vi "Big_LED_control.vi"() -> ()   [LabVIEW 2018]
uses:
  <instrlib>/niDMM/nidmm.llb/niDMM Function.ctl
  <instrlib>/niDMM/nidmm.llb/niDMM Resolution in Digits.ctl
  <instrlib>/niDCPower/nidcpower.llb/niDCPower Measurement Type.ctl
  <instrlib>/niDMM/nidmm.llb/niDMM Configure Measurement Digits.vi
  <vilib>/Instr/_visa.llb/VISA Configure Serial Port (Instr).vi
panel:
  in  "Записать":bool
  in  "Command":string="led_on"
  in  "Tab Control":enum32{"Рабочая область", "Служебная область"}(tab)
  in  "POWER":bool
  in  "Стоп":bool
  in  "Resource Name":refnum<k15>="PXI1Slot2" caption="Источник питания"
  in  "Амперметр":refnum<k15>="PXI1Slot5" caption="NI DMM 1"
  in  "V_MB, V":dbl=5.0 caption="voltage level" format="%_6p"
  in  "curlim_V_MB, A":dbl=0.3 caption="current limit" format="%_6p"
  in  "curlim_V_RESERVE, A":dbl=0.1 caption="current limit" min=0.01 format="%_6p"
  out "currentmes_V_MB, A":dbl caption="measurement" format="%_6g"
  out "currentmes_V_RESERVE, A":dbl caption="measurement" format="%_6g"
  in  "V_RESERVE, V":dbl caption="voltage level" format="%_6p"
  out "chart_2":dbl(graph)=8.556104343922883e-07
  out "chart_0":dbl(graph)=5.42616690347781e-05 caption="Waveform Chart 5"
  in  "curlim_V_LED, A":dbl=0.01 caption="current limit" min=0.01 format="%_6p"
  in  "V_LED, V":dbl=2.000000000000001 caption="voltage level" format="%_6p"
  out "chart_1":dbl(graph)=2.456762028615791e-06 caption="Waveform Chart 5"
  out "currentmes_V_LED, A":dbl caption="measurement" format="%_6g"
  in  "NI DMM 1 Current Range 3":string(combo)="1" caption="Range"
  in  "NI DMM 1 units 3":string(combo)="1000" caption="Units"
  out "Current Char":dbl(graph)=0.013612861948786303
  out "Current":dbl format="%_6g"
  in  "Arduino":refnum<visa-resource-name>="COM14"
  out "Сегменты":bool[](array[boolean])
  in  "Вольтметр":refnum<k15>="PXI1Slot5" caption="NI DMM 1"
  in  "NI DMM 1 Voltage Range 4":string(combo)="-1" caption="Range"
  out "Voltage Char":dbl(graph)=0.013612861948786303
  in  "NI DMM 1 units 4":string(combo)="1" caption="Units"
  out "Voltage":dbl format="%_6g"
  out "Тип индикатора":string
  out "Разряд":dbl
  out "+/-":bool
  out "Power off":bool
  # "V_MB 5 В\nогрничение 300 м\n\nV_LED 2,1 В\nограничение 200 м"
  # "1. каждый сегмент включаем по отдельности, резистором постраиваем ток до 10 мА\n2. напряжение V_LED при этом не меняется\n3. в такоом положении промеряем сегменты по отдельности\n4. для промера всего индикатора сразу подстраиваем напряжение при неизменном положении резисторов\n5. ток всех индикаторов = ток одного сегмента (10 мА) * число сегментов (15)\n6. добиваемся этого увеличением V_LED"
  # "единицы мА\nrange 1 А"
  # "единицы В\nrange AUTO"
  # "24.063\n\n     I          U\n20 мА  1.3 В\n20 мА  1.4 В\n 7 мА   1.15 В"
  # "24.064\n\n     I          U\n10 мА  2 В\n10 мА  2.15 В\n 7 мА   1.9 В"
  # "Р1:  +25°C\nР2:  - 60°C\nР3:  +85°C"
  # "j"
  # "c"
  # "d"
  # "e"
  # "g"
  # "h"
  # "a"
  # "b"
  # "f"
  # "k"
  # "L"
  # "m"
  # "n"
  # "p"
  # "dp"
  # "all"
  # "необходимо выдерживать 1 с между нажатиями кнопок"
  # "регулировать ток в зависимости от температуры.\nс ростом температуры растет ток.\nпид-регулятор??"
  # "\"опрашивать кнопки не чаще, чем раз в секунду. сейчас кликать можно чаще, они загорятся, но ничего не произойдет\""
  # "автоматизировать подбор напряжения по известному максимальному напряжению и току. ОС по току сегмента"
  # "регклировка суммарного тока через инлдикатор"
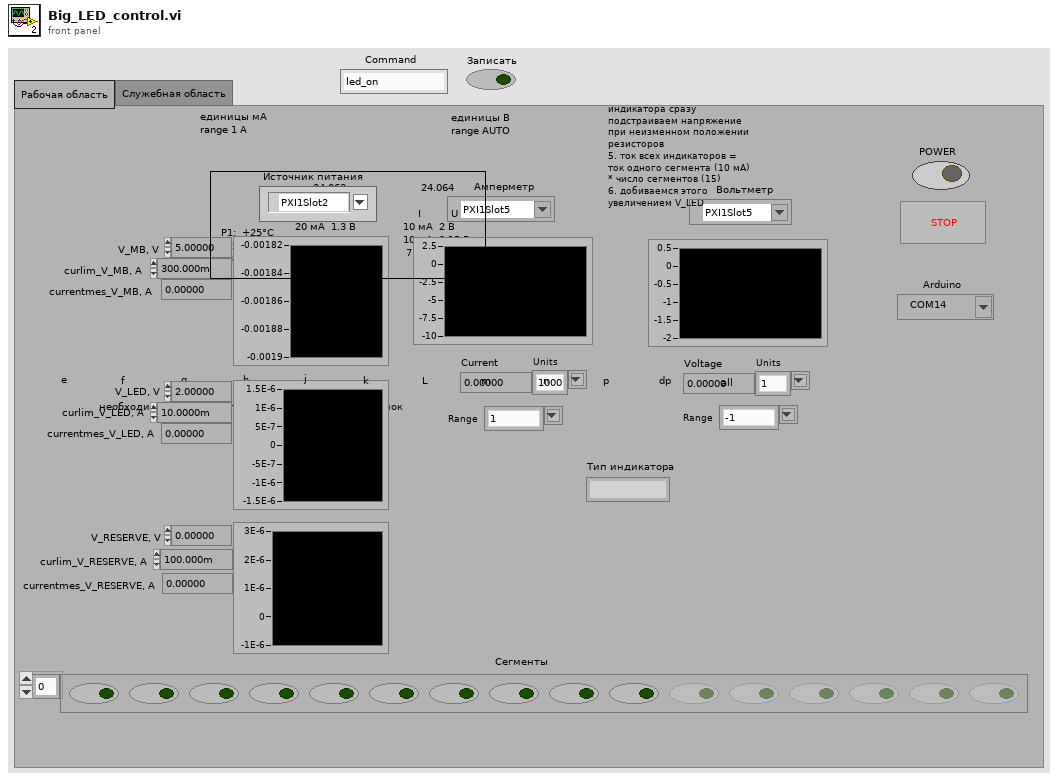
[diagram p1: front panel]
types:
  T1 = typedef "niDMM Function.ctl" = enum16{"DC Volts", "AC Volts", "DC Current", "AC Current", "2-wire Resistance", "4-wire Resistance", "Diode", "Frequency", "Period", "AC Volts DC Coupled", "Capacitance", "Inductance", "Temperature"}
  T2 = typedef "niDMM Resolution in Digits.ctl" = dbl
  T3 = typedef "niDCPower Measurement Type.ctl" = i32
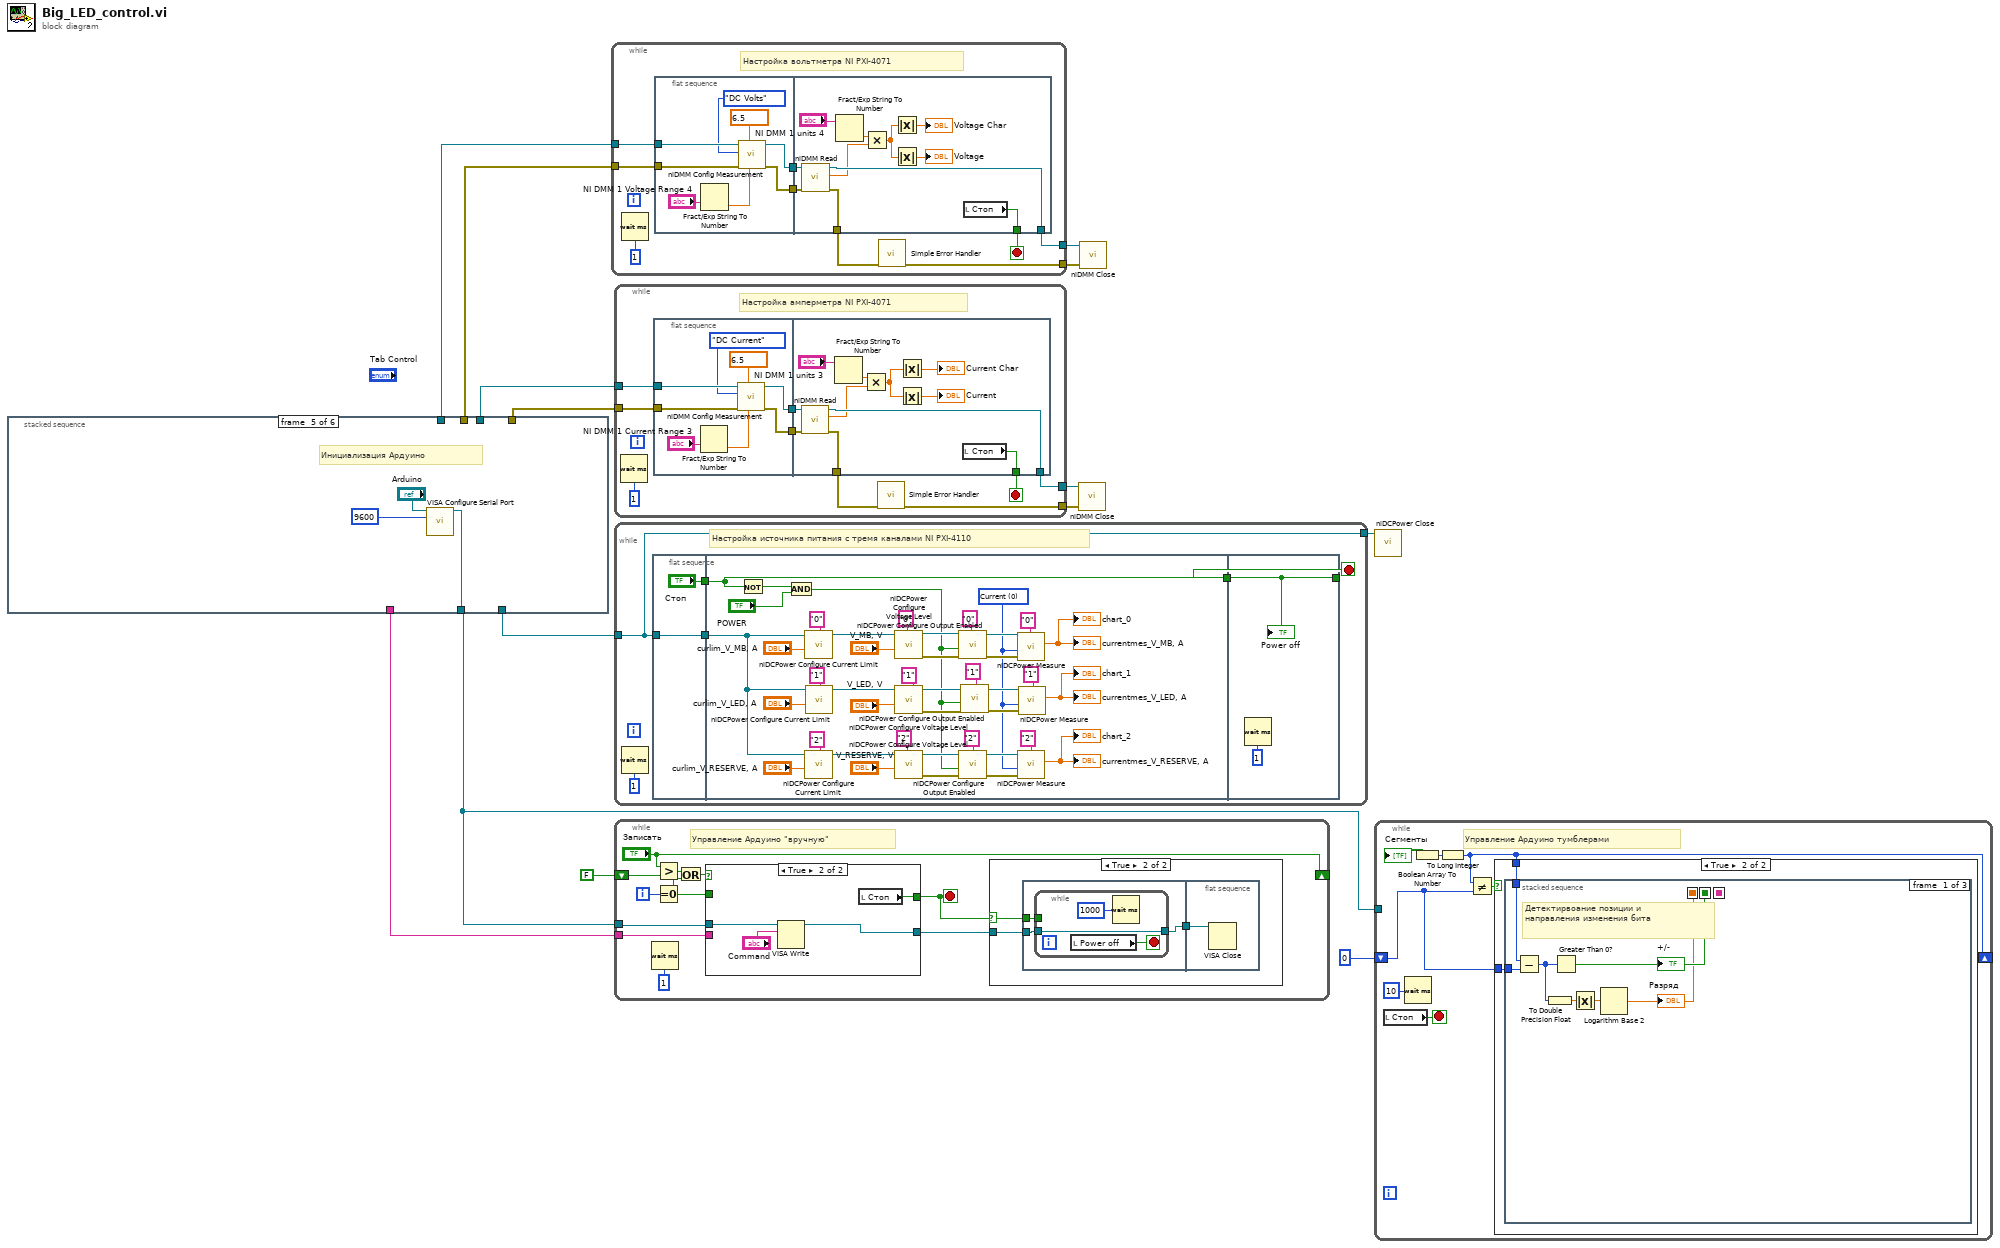
[diagram p0: block diagram]
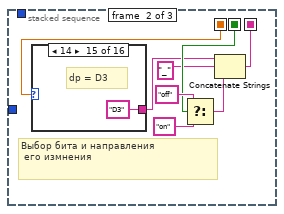
[diagram p3: hidden frame]
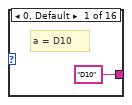
[diagram p4: hidden frame]
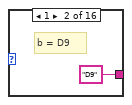
[diagram p5: hidden frame]
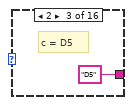
[diagram p6: hidden frame]
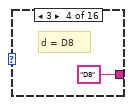
[diagram p7: hidden frame]
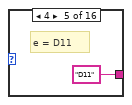
[diagram p8: hidden frame]
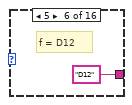
[diagram p9: hidden frame]
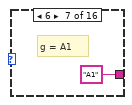
[diagram p10: hidden frame]
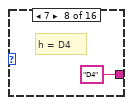
[diagram p11: hidden frame]
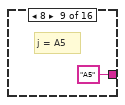
[diagram p12: hidden frame]
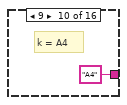
[diagram p13: hidden frame]
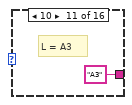
[diagram p14: hidden frame]
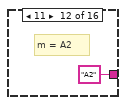
[diagram p15: hidden frame]
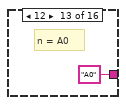
[diagram p16: hidden frame]
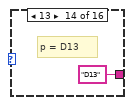
[diagram p17: hidden frame]
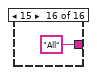
[diagram p18: hidden frame]
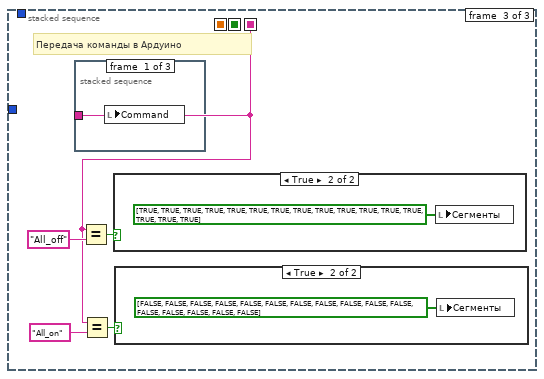
[diagram p19: hidden frame]
diagram:
  n1 = stacked-sequence {
    tunnel: [_ _ _ w27 _ _] -> w11
    tunnel: [_ w21 _ _ _ _] -> w14
    tunnel: [_ w20 _ _ _ _] -> w13
    tunnel: [_ _ _ _ w31 _] -> w8
    tunnel: [_ _ _ _ _ w34] -> w7
    tunnel: [_ _ w24 _ _ _] -> w6
    tunnel: [_ _ w23 _ _ _] -> w5
    frame #0 {
      w17 = 0.0 ("currentmes_2")
      w16 = FALSE ("Стоп")
      # "Обнуление переменных"
      n2 = local write "Стоп"(w16) -> ()
      n3 = local write "+/-"(w16) -> ()
      n4 = local write "POWER"(w16) -> ()
      n5 = local write "Сегменты"(bool[] [FALSE, FALSE, FALSE, FALSE, FALSE, FALSE, FALSE, FALSE, FALSE, FALSE, FALSE, FALSE, FALSE, FALSE, FALSE, FALSE, FALSE, FALSE] ("Сегменты")) -> ()
      n6 = local write "currentmes_V_MB, A"(w17) -> ()
      n7 = local write "currentmes_V_LED, A"(w17) -> ()
      n8 = local write "currentmes_V_RESERVE, A"(w17) -> ()
      n9 = local write "Разряд"(w17) -> ()
      n10 = local write "Command"("zero" ("Command 2")) -> ()
      n11 = local write "Current"(w17) -> ()
    }
    frame #1 {
      # "Инициализация амперметра"
      n12 = call <instrlib>:"niDMM Initialize.vi"("Instrument Descriptor"="Амперметр") -> ("error out"=w21:errorcluster, "instrument handle out"=w20:refnum<k15>)  [unwired: 9 in]
    }
    frame #2 {
      # "Инициализация вольтметра"
      n13 = call <instrlib>:"niDMM Initialize.vi"("Instrument Descriptor"="Вольтметр") -> ("error out"=w23:errorcluster, "instrument handle out"=w24:refnum<k15>)  [unwired: 9 in]
    }
    frame #3 {
      # "Инициализация источника питания"
      n14 = call <instrlib>:"niDCPower Initialize.vi"("resource name"="Resource Name") -> ("error out"=w26:errorcluster, "instrument handle out"=w28:refnum<k15>)  [unwired: 3 in, 6 out]
      n15 = call <instrlib>:"niDCPower Configure Voltage Level.vi"("error in (no error)"=w26, "voltage level"=0.0, "channel name"="0,1,2", "instrument handle"=w28) -> ("instrument handle out"=w27:refnum<k15>)  [unwired: 6 in, 1 out]
    }
    frame #4 {
      # "Инициализация Ардуино"
      n16 = call-poly "VISA Configure Serial Port"("VISA resource name"="Arduino", "baud rate (9600)"=u32 9600) -> ("VISA resource name out"=w31:refnum<visa-resource-name>)  [unwired: 12 in, 1 out]
    }
    frame #5 {
      # "Всплывающее окно\nкакой индикатор?\nОА/ОК"
      n17 = call "Begin.vi"() -> ("String"=w34:string)  [unwired: 8 in]
      "Тип индикатора" <- w34
      n18 = local write "Command"(w34) -> ()
    }
  }
  n19 = while {
    tunnel: [w41] -> w3
    tunnel: w6 -> [w39]
    tunnel: w5 -> [w38]
    tunnel: [w35] -> w4
    stop <- w37 stop-if-true
    # "Настройка вольтметра NI PXI-4071"
    n20 = Wait (ms)(milliseconds to wait=u32 1) -> ()  [unwired: 1 out]
    n21 = flat-sequence {
      tunnel: [w48] -> w43
      tunnel: w39 -> [w46]
      tunnel: w38 -> [w50]
      tunnel: [w47] -> w42
      tunnel: w43 -> [w59]
      tunnel: w42 -> [w62]
      tunnel: [w58] -> w37
      tunnel: [w57] -> w35
      tunnel: [w56] -> w36
      frame #0 {
        w44 = T2 6.5 items=["3 1/2"=3.5, "4 1/2"=4.5, "5 1/2"=5.5, "6 1/2"=6.5, "7 1/2"=7.5] ("Resolution in Digits")
        n22 = Fract/Exp String To Number(string="NI DMM 1 Voltage Range 4") -> (number=w49:dbl)  [unwired: 3 in, 1 out]
        n23 = call-poly <instrlib>:"niDMM Config Measurement.vi"("Range"=w49, "Resolution in Digits"=w44, "error in (no error)"=w50, "Function"=niDMM_Function."DC Volts" ("Measurement Type"), "instrument handle"=w46) -> ("error out"=w47:errorcluster, "instrument handle out"=w48:refnum<k15>)  [unwired: 5 in]
      }
      frame #1 {
        n24 = call <instrlib>:"niDMM Read.vi"("error in (no error)"=w62, "instrument handle"=w59) -> ("error out"=w56:errorcluster, "Measurement"=w54:dbl, "instrument handle out"=w57:refnum<k15>)  [unwired: 7 in]
        n25 = Fract/Exp String To Number(string="NI DMM 1 units 4") -> (number=w60:dbl)  [unwired: 3 in, 1 out]
        n26 = Multiply(x=w60, y=w54) -> (x*y=w52:dbl)
        n27 = Absolute Value(x=w52) -> (abs(x)=→"Voltage Char":dbl)
        n28 = Absolute Value(x=w52) -> (abs(x)=→"Voltage":dbl)
        n29 = local read "Стоп"() -> (w58:bool)
      }
    }
    n30 = call <vilib>:"Simple Error Handler.vi"("error in (no error)"=w36) -> ("error out"=w41:errorcluster)  [unwired: 1 in, 7 out]
  }
  n31 = while {
    tunnel: w11 -> [w64]
    tunnel: [w64] -> w10
    stop <- w65 stop-if-true
    # "Настройка источника питания с тремя каналами NI PXI-4110"
    n32 = Wait (ms)(milliseconds to wait=u32 1) -> ()  [unwired: 1 out]
    n33 = flat-sequence {
      tunnel: w64 -> [w70]
      tunnel: [w70] -> w67
      tunnel: ["Стоп"] -> w66
      tunnel: w67 -> [w78]
      tunnel: w66 -> [w112]
      tunnel: [w112] -> w63
      tunnel: [w114] -> w65
      tunnel: w63 -> [w114]
      frame #0 {
      }
      frame #1 {
        w77 = T3 0 items=["Current", "Voltage"] ("measurement type")
        n34 = Not(x=w112) -> (.not. x?=w111:bool)
        n35 = And(x=w111, y="POWER") -> (x .and. y?=w73:bool)
        n36 = call <instrlib>:"niDCPower Configure Current Limit.vi"("current limit"="curlim_V_MB, A", "channel name"="0", "instrument handle"=w78) -> ("instrument handle out"=w97:refnum<k15>)  [unwired: 7 in, 1 out]
        n37 = call <instrlib>:"niDCPower Configure Current Limit.vi"("current limit"="curlim_V_RESERVE, A", "channel name"="2", "instrument handle"=w78) -> ("instrument handle out"=w96:refnum<k15>)  [unwired: 7 in, 1 out]
        n38 = call <instrlib>:"niDCPower Configure Current Limit.vi"("current limit"="curlim_V_LED, A", "channel name"="1", "instrument handle"=w78) -> ("instrument handle out"=w105:refnum<k15>)  [unwired: 7 in, 1 out]
        n39 = call <instrlib>:"niDCPower Configure Voltage Level.vi"("voltage level"="V_MB, V", "channel name"="0", "instrument handle"=w97) -> ("error out"=w102:errorcluster, "instrument handle out"=w99:refnum<k15>)  [unwired: 7 in]
        n40 = call <instrlib>:"niDCPower Configure Voltage Level.vi"("voltage level"="V_LED, V", "channel name"="1", "instrument handle"=w105) -> ("error out"=w108:errorcluster, "instrument handle out"=w106:refnum<k15>)  [unwired: 7 in]
        n41 = call <instrlib>:"niDCPower Configure Voltage Level.vi"("voltage level"="V_RESERVE, V", "channel name"="2", "instrument handle"=w96) -> ("error out"=w101:errorcluster, "instrument handle out"=w100:refnum<k15>)  [unwired: 7 in]
        n42 = call <instrlib>:"niDCPower Configure Output Enabled.vi"("error in (no error)"=w102, "output enabled"=w73, "channel name"="0", "instrument handle"=w99) -> ("error out"=w92:errorcluster, "instrument handle out"=w93:refnum<k15>)  [unwired: 6 in]
        n43 = call <instrlib>:"niDCPower Configure Output Enabled.vi"("error in (no error)"=w101, "output enabled"=w73, "channel name"="2", "instrument handle"=w100) -> ("error out"=w91:errorcluster, "instrument handle out"=w90:refnum<k15>)  [unwired: 6 in]
        n44 = call <instrlib>:"niDCPower Configure Output Enabled.vi"("error in (no error)"=w108, "output enabled"=w73, "channel name"="1", "instrument handle"=w106) -> ("error out"=w109:errorcluster, "instrument handle out"=w107:refnum<k15>)  [unwired: 6 in]
        n45 = call <instrlib>:"niDCPower Measure.vi"("error in (no error)"=w92, "measurement type"=w77, "channel name"="0", "instrument handle"=w93) -> ("measurement"=→"currentmes_V_MB, A" →"chart_0":dbl)  [unwired: 5 in, 2 out]
        n46 = call <instrlib>:"niDCPower Measure.vi"("error in (no error)"=w91, "measurement type"=w77, "channel name"="2", "instrument handle"=w90) -> ("measurement"=→"currentmes_V_RESERVE, A" →"chart_2":dbl)  [unwired: 5 in, 2 out]
        n47 = call <instrlib>:"niDCPower Measure.vi"("error in (no error)"=w109, "measurement type"=w77, "channel name"="1", "instrument handle"=w107) -> ("measurement"=→"chart_1" →"currentmes_V_LED, A":dbl)  [unwired: 5 in, 2 out]
      }
      frame #2 {
        n48 = Wait (ms)(milliseconds to wait=u32 1) -> ()  [unwired: 1 out]
        "Power off" <- w114
      }
    }
  }
  n49 = while {
    tunnel: [w121] -> w1
    tunnel: w13 -> [w119]
    tunnel: w14 -> [w118]
    tunnel: [w115] -> w2
    stop <- w117 stop-if-true
    # "Настройка амперметра NI PXI-4071"
    n50 = Wait (ms)(milliseconds to wait=u32 1) -> ()  [unwired: 1 out]
    n51 = flat-sequence {
      tunnel: [w128] -> w123
      tunnel: w119 -> [w126]
      tunnel: w118 -> [w130]
      tunnel: [w127] -> w122
      tunnel: w123 -> [w139]
      tunnel: w122 -> [w142]
      tunnel: [w138] -> w117
      tunnel: [w137] -> w115
      tunnel: [w136] -> w116
      frame #0 {
        w124 = T2 6.5 items=["3 1/2"=3.5, "4 1/2"=4.5, "5 1/2"=5.5, "6 1/2"=6.5, "7 1/2"=7.5] ("Resolution in Digits")
        n52 = Fract/Exp String To Number(string="NI DMM 1 Current Range 3") -> (number=w129:dbl)  [unwired: 3 in, 1 out]
        n53 = call-poly <instrlib>:"niDMM Config Measurement.vi"("Range"=w129, "Resolution in Digits"=w124, "error in (no error)"=w130, "Function"=niDMM_Function."DC Current" ("Measurement Type"), "instrument handle"=w126) -> ("error out"=w127:errorcluster, "instrument handle out"=w128:refnum<k15>)  [unwired: 5 in]
      }
      frame #1 {
        n54 = call <instrlib>:"niDMM Read.vi"("error in (no error)"=w142, "instrument handle"=w139) -> ("error out"=w136:errorcluster, "Measurement"=w134:dbl, "instrument handle out"=w137:refnum<k15>)  [unwired: 7 in]
        n55 = Fract/Exp String To Number(string="NI DMM 1 units 3") -> (number=w140:dbl)  [unwired: 3 in, 1 out]
        n56 = Multiply(x=w140, y=w134) -> (x*y=w132:dbl)
        n57 = Absolute Value(x=w132) -> (abs(x)=→"Current Char":dbl)
        n58 = Absolute Value(x=w132) -> (abs(x)=→"Current":dbl)
        n59 = local read "Стоп"() -> (w138:bool)
      }
    }
    n60 = call <vilib>:"Simple Error Handler.vi"("error in (no error)"=w116) -> ("error out"=w121:errorcluster)  [unwired: 1 in, 7 out]
  }
  n61 = while {
    tunnel: w8 -> [w150]
    shift-right: ["Записать"] -> _
    shift-left: FALSE ("Записать") -> [w152]
    tunnel: w7 -> [w148]
    i -> [w149]
    stop <- w144 stop-if-true
    # "Управление Ардуино \"вручную\""
    n62 = Wait (ms)(milliseconds to wait=u32 1) -> ()  [unwired: 1 out]
    n63 = Greater?(x="Записать", y=w152) -> (0:w146:bool)
    n64 = Equal To 0?(x=w149) -> (x = 0?=w145:bool)
    n65 = Or(x=w146, y=w145) -> (x .or. y?=w147:bool)
    n66 = case shown="True" w147 {
      tunnel: w150 -> [w164 w169]
      tunnel: [w165 w168] -> w144
      tunnel: w148 -> [_ _]
      tunnel: w145 -> [_ _]
      tunnel: [w164 w166] -> w143
      frame False {
        n67 = local read "Стоп"() -> (w165:bool)
      }
      frame True {
        n68 = VISA Write(VISA resource name=w169, write buffer="Command") -> (VISA resource name out=w166:refnum<visa-resource-name>)  [unwired: 1 in, 2 out]
        n69 = local read "Стоп"() -> (w168:bool)
      }
    }
    n70 = case shown="True" w144 {
      selector: w144 -> [_ w154]
      tunnel: w143 -> [_ w156]
      frame False {
      }
      frame True {
        n71 = flat-sequence {
          tunnel: w156 -> [w159]
          tunnel: [w158] -> w155
          tunnel: w154 -> [w157]
          tunnel: w155 -> [w163]
          frame #0 {
            n72 = while {
              tunnel: w159 -> [w162]
              tunnel: [w162] -> w158
              tunnel: w157 -> [_]
              stop <- w160 stop-if-true
              n73 = local read "Power off"() -> (w160:bool)
              n74 = Wait (ms)(milliseconds to wait=u32 1000) -> ()  [unwired: 1 out]
            }
          }
          frame #1 {
            n75 = VISA Close(VISA resource name=w163) -> ()  [unwired: 1 in, 1 out]
          }
        }
      }
    }
  }
  n76 = call <instrlib>:"niDMM Close.vi"("error in (no error)"=w1, "instrument handle"=w2) -> ()  [unwired: 9 in, 1 out]
  n77 = call <instrlib>:"niDMM Close.vi"("error in (no error)"=w3, "instrument handle"=w4) -> ()  [unwired: 9 in, 1 out]
  n78 = call <instrlib>:"niDCPower Close.vi"("instrument handle"=w10) -> ()  [unwired: 10 in, 1 out]
  n79 = while {
    shift-right: [w171] -> _
    shift-left: i16 0 -> [w172]
    tunnel: w8 -> [_]
    stop <- w176 stop-if-true
    # "Управление Ардуино тумблерами"
    n80 = local read "Стоп"() -> (w176:bool)
    n81 = Wait (ms)(milliseconds to wait=u32 10 ("millisecond timer value")) -> ()  [unwired: 1 out]
    n82 = Boolean Array To Number(Boolean array="Сегменты") -> (number=w170:u32)
    n83 = To Long Integer(number=w170) -> (32bit integer=w171:i32)
    n84 = Not Equal?(x=w171, y=w172) -> (x != y?=w173:bool)
    n85 = case shown="True" w173 {
      tunnel: w171 -> [_ w177]
      tunnel: w172 -> [_ w178]
      frame False {
      }
      frame True {
        n86 = stacked-sequence {
          seq-local: [w181 _ _] -> [_ w191 _]
          seq-local: [w179 _ _] -> [_ w186 _]
          seq-local: [_ w187 _] -> [_ _ w211]
          tunnel: w177 -> [w183 _ _]
          tunnel: w178 -> [w182 _ _]
          frame #0 {
            # "Детектирвоание позиции и\nнаправления изменения бита"
            n87 = Subtract(x=w183, y=w182) -> (x-y=w184:i32)
            n88 = To Double Precision Float(number=w184) -> (double precision float=w185:dbl)
            n89 = Greater Than 0?(x=w184) -> (x > 0?=w181:bool)
            "+/-" <- w181
            n90 = Absolute Value(x=w185) -> (abs(x)=w180:dbl)
            n91 = Logarithm Base 2(1:w180) -> (0:w179:dbl)
            "Разряд" <- w179
          }
          frame #1 {
            # "Выбор бита и направления\n его измнения"
            n92 = case shown="14" w186 {
              tunnel: ["D10" "D9" "D5" "D8" "D11" "D12" "A1" "D4" "A5" "A4" "A3" "A2" "A0" "D13" "D3" "All"] -> w189
              frame 0, Default {
                # "a = D10"
              }
              frame 1 {
                # "b = D9"
              }
              frame 2 {
                # "c = D5"
              }
              frame 3 {
                # "d = D8"
              }
              frame 4 {
                # "e = D11"
              }
              frame 5 {
                # "f = D12"
              }
              frame 6 {
                # "g = A1"
              }
              frame 7 {
                # "h = D4"
              }
              frame 8 {
                # "j = A5"
              }
              frame 9 {
                # "k = A4"
              }
              frame 10 {
                # "L = A3"
              }
              frame 11 {
                # "m = A2"
              }
              frame 12 {
                # "n = A0"
              }
              frame 13 {
                # "p = D13"
              }
              frame 14 {
                # "dp = D3"
              }
              frame 15 {
              }
            }
            n93 = Select(t="off", s=w191, f="on") -> (s? t:f=w188:string)
            n94 = Concatenate Strings(w189, "_" ("string"), w188) -> (w187:string)
          }
          frame #2 {
            # "Передача команды в Ардуино"
            n95 = stacked-sequence {
              tunnel: w211 -> [w217 _ _]
              frame #0 {
                n96 = local write "Command"(w217) -> ()
              }
              frame #1 {
                n97 = local write "Записать"(TRUE ("Записать")) -> ()
                n98 = Wait (ms)(milliseconds to wait=u32 1000) -> ()  [unwired: 1 out]
              }
              frame #2 {
                n99 = local write "Записать"(FALSE ("Записать")) -> ()
                n100 = Wait (ms)(milliseconds to wait=u32 1000) -> ()  [unwired: 1 out]
              }
            }
            n101 = Equal?(x=w211, y="All_off") -> (x = y?=w214:bool)
            n102 = Equal?(x=w211, y="All_on") -> (x = y?=w212:bool)
            n103 = case shown="True" w214 {
              frame False {
              }
              frame True {
                n104 = local write "Сегменты"(bool[] [TRUE, TRUE, TRUE, TRUE, TRUE, TRUE, TRUE, TRUE, TRUE, TRUE, TRUE, TRUE, TRUE, TRUE, TRUE, TRUE] ("Сегменты")) -> ()
              }
            }
            n105 = case shown="True" w212 {
              frame False {
              }
              frame True {
                n106 = local write "Сегменты"(bool[] [FALSE, FALSE, FALSE, FALSE, FALSE, FALSE, FALSE, FALSE, FALSE, FALSE, FALSE, FALSE, FALSE, FALSE, FALSE, FALSE] ("Сегменты")) -> ()
              }
            }
          }
        }
      }
    }
  }
